vi "choose_crystals.vi"(5 "ROI Size":T2, 7 "Parameters":T3, 8 "Error In":errorcluster, 9 "Xi":T4, 10 "Sample":string, 11 "File Path":path) -> (0 "Error Out":errorcluster, 3 "ROIs Out":T1(array[cluster]))   [LabVIEW 2019]
uses:
  xi_angles_enum_typedef.ctl
  parameters_cluster_typedef.ctl
  sections_roi_size_enum_typedef.ctl
  choose_crystals_states_enum_typedef.ctl
  <vilib>/vision/NI_Vision_Development_Module.lvlib
panel:
  in  "Done":bool
  in  "Frame":i32(slide) scale=0.0..3.0
  in  "X Value":sgl format="%.2f"
  in  "Operator":T5(ring)
  out "Image":T6(plugin-control)
  # "Choose Crystals"
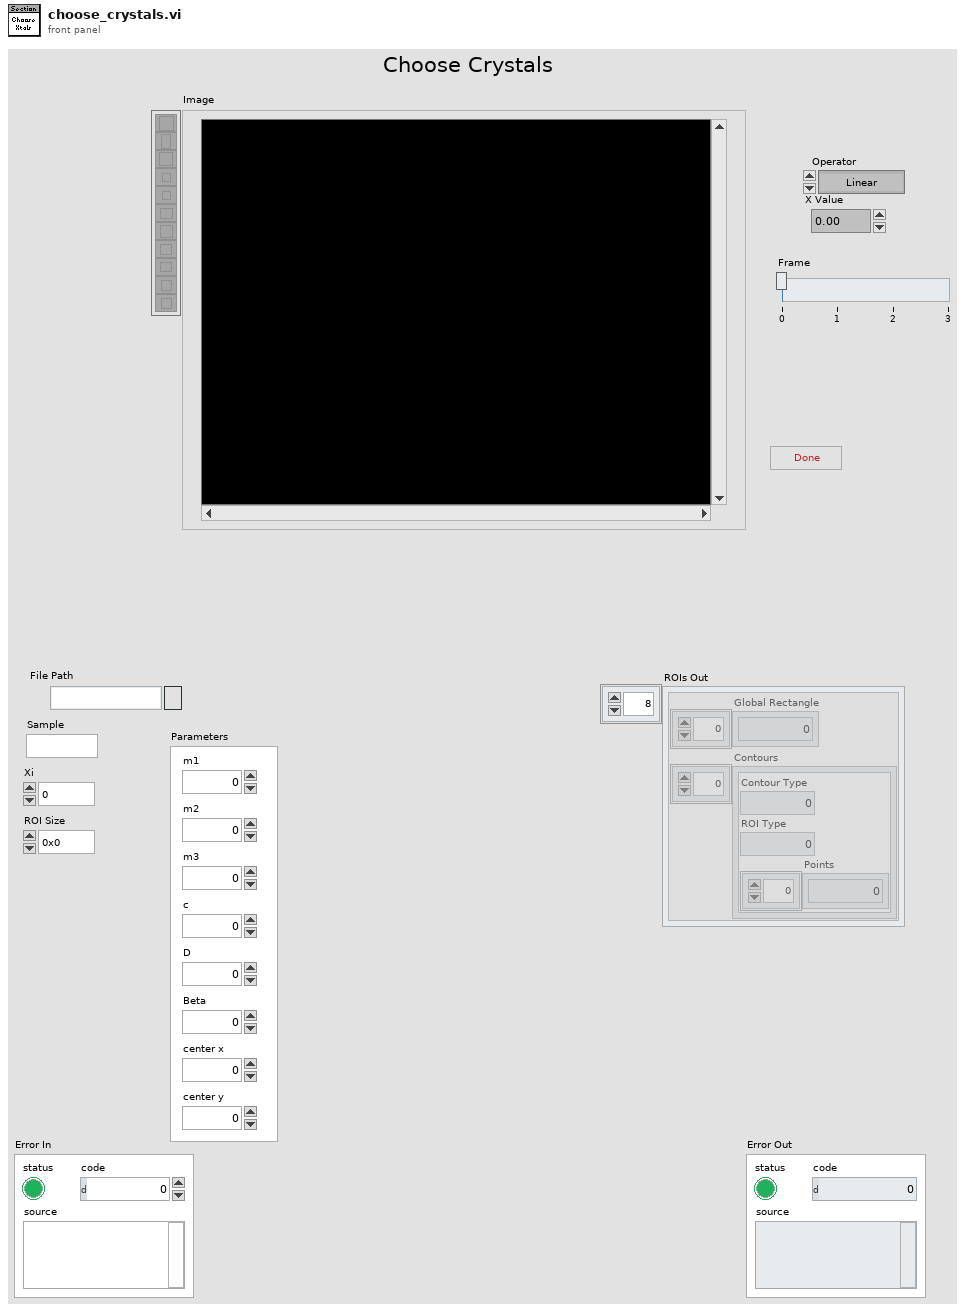
[diagram p1: front panel]
types:
  T1 = cluster{"Global Rectangle":i32[], "Contours":cluster{"Contour Type":u32, "ROI Type":u32, "Points":i32[]}[]}[]
  T2 = typedef "sections_roi_size_enum_typedef.ctl" = enum16{"0x0", "1x1", "2x2", "3x3", "4x4", "5x5", "6x6"}
  T3 = typedef "parameters_cluster_typedef.ctl" = cluster{"m1":dbl, "m2":dbl, "m3":dbl, "c":dbl, "D":dbl, "Beta":dbl, "center x":dbl, "center y":dbl}
  T4 = typedef "xi_angles_enum_typedef.ctl" = enum16{"0", "45"}
  T5 = enum32{"Linear", "Log", "Exp", "Square", "Square root", "Power X", "Power 1/X"}
  T6 = typedef "IMAQ Image.ctl" = refnum<image>
  T7 = typedef "choose_crystals_states_enum_typedef.ctl" = enum16{"Initialize", "Wait", "Shutdown", "Plot Image", "Process"}
  T8 = cluster{"Global Rectangle":i32[], "Contours":cluster{"Contour Type":u32, "ROI Type":u32, "Points":i32[]}[]}
  T9 = typedef "ROI Descriptor" = cluster{"Global Rectangle":i32[], "Contours":cluster{"ID":enum32{"External", "Internal"}, "Type":u32, "Coordinates":i32[]}[]}
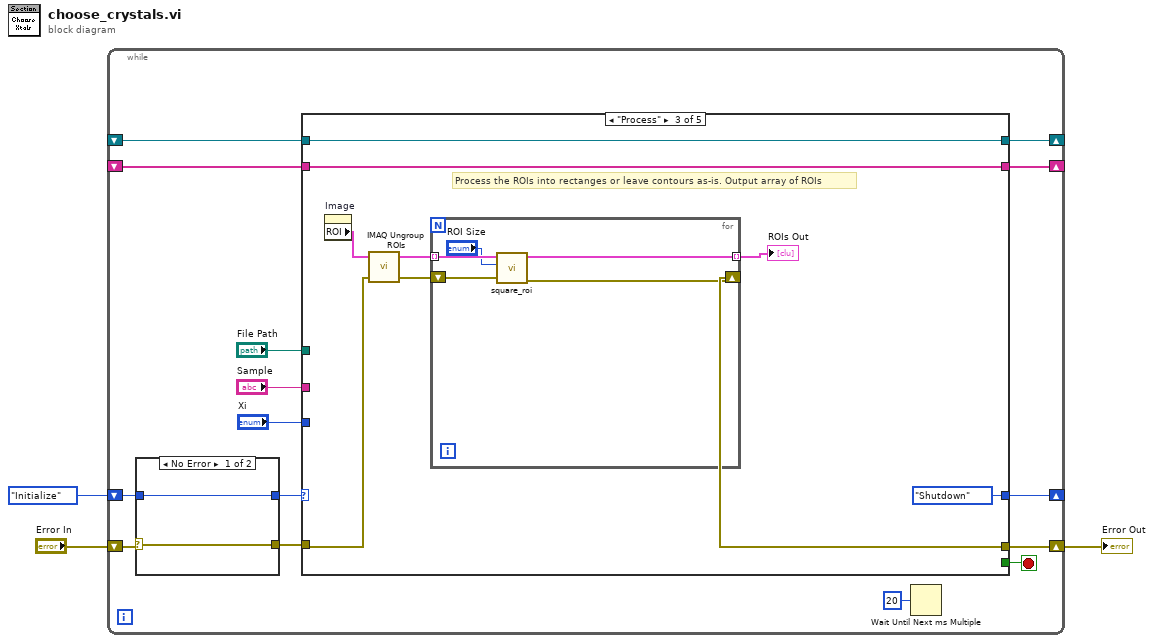
[diagram p0: block diagram]
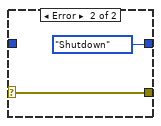
[diagram p2: hidden frame]
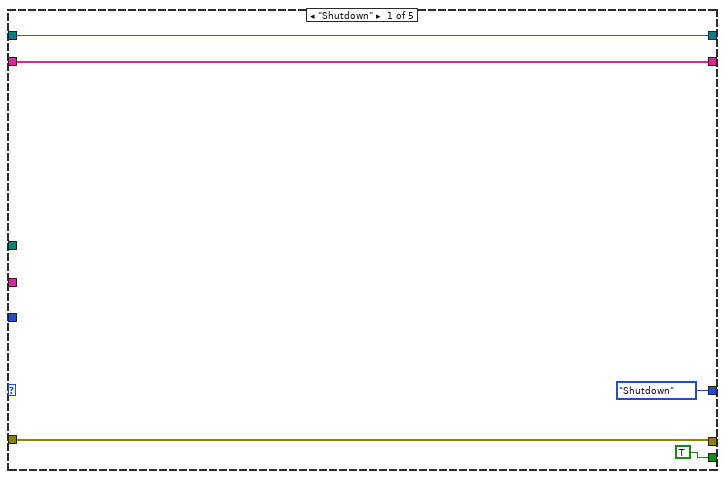
[diagram p3: hidden frame]
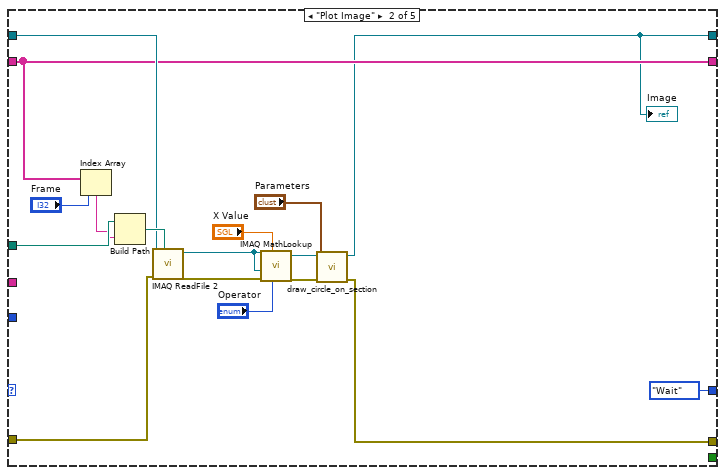
[diagram p4: hidden frame]
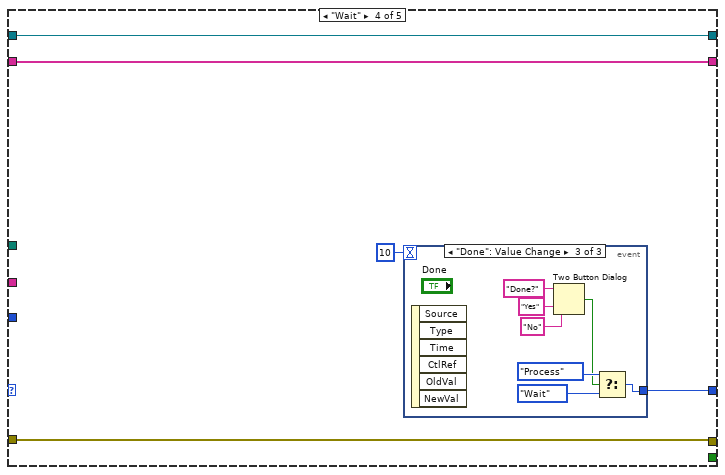
[diagram p5: hidden frame]
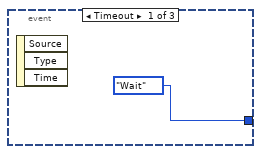
[diagram p6: hidden frame]
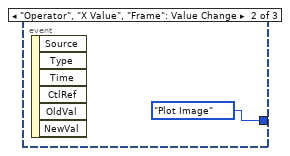
[diagram p7: hidden frame]
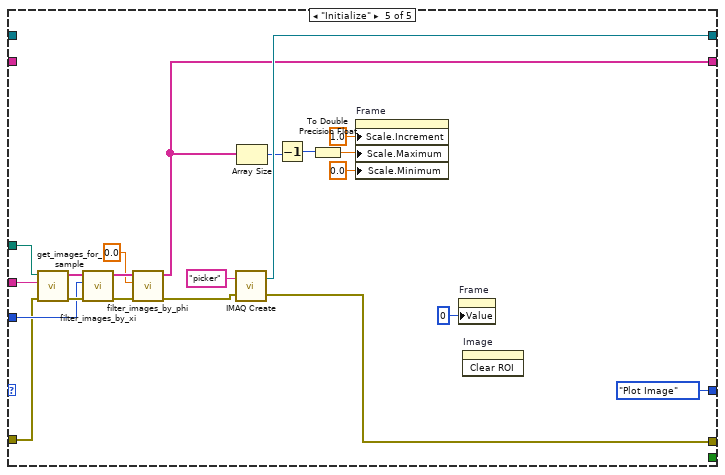
[diagram p8: hidden frame]
diagram:
  n1 = while {
    shift-right: [w14] -> _
    shift-left: choose_crystals_states_enum_typedef."Initialize" -> [w17]
    shift-right: [w13] -> w1
    shift-left: "Error In" -> [w16]
    shift-right: [w7] -> _
    shift-left: _ -> [w6]
    shift-right: [w5] -> _
    shift-left: _ -> [w4]
    stop <- w11 stop-if-true
    n2 = case shown="No Error" w16 {
      selector: w16 -> [w19 w22]
      tunnel: [w20 choose_crystals_states_enum_typedef."Shutdown"] -> w18
      tunnel: w17 -> [w20 _]
      tunnel: [w19 w22] -> w15
      frame No Error {
      }
      frame Error {
      }
    }
    n3 = case shown="\"Process\"" w18 {
      tunnel: w15 -> [w26 w37 w49 w61 w84]
      tunnel: [choose_crystals_states_enum_typedef."Shutdown" choose_crystals_states_enum_typedef."Wait" choose_crystals_states_enum_typedef."Shutdown" w62 choose_crystals_states_enum_typedef."Plot Image"] -> w14
      tunnel: [w26 w29 w45 w61 w83] -> w13
      tunnel: [TRUE _ _ _ _] -> w11
      tunnel: "File Path" -> [_ w40 _ _ w92]
      tunnel: "Sample" -> [_ _ _ _ w91]
      tunnel: "Xi" -> [_ _ _ _ w86]
      tunnel: [w23 w35 w51 w59 w74] -> w7
      tunnel: w6 -> [w23 w35 w51 w59 _]
      tunnel: [w24 w28 w52 w60 w80] -> w5
      tunnel: w4 -> [w24 w36 w52 w60 _]
      frame "Shutdown" {
      }
      frame "Plot Image" {
        n4 = Index Array(array=w35, index="Frame") -> (element=w39:string)
        n5 = Build Path(base path=w40, name or relative path=w39) -> (appended path=w38:path)
        n6 = call "IMAQ ReadFile 2"("File Path"=w38, "error in (no error)"=w37, "Image"=w36) -> ("error out"=w33:errorcluster, "Image Out"=w34:T6)  [unwired: 4 in, 3 out]
        n7 = call "IMAQ MathLookup"("Operator"="Operator", "X Value"="X Value", "error in (no error)"=w33, "Image Dst"=w34, "Image Src"=w34) -> ("error out"=w30:errorcluster, "Image Dst Out"=w32:T6)  [unwired: 5 in]
        n8 = call "draw_circle_on_section.vi"("Error In"=w30, "Parameters"="Parameters", "Image Src"=w32) -> ("Error Out"=w29:errorcluster, "Image Dst Out"=w28:T6)  [unwired: 7 in]
        "Image" <- w28
      }
      frame "Process" {
        # "Process the ROIs into rectanges or leave contours as-is. Output array of ROIs"
        n9 = property on="Image" class="ImageControl"() -> ("ROI"=w50:T8)  [unwired: 2 in, 2 out]
        n10 = call "IMAQ Ungroup ROIs"("error in (no error)"=w49, "ROI Descriptor"=w50) -> ("error out"=w47:errorcluster, "ROI Descriptors out"=w48:T9[])  [unwired: 2 in]
        n11 = for {
          tunnel: w48 -> [w58] mode=indexing
          shift-right: [w55] -> w45
          shift-left: w47 -> [w57]
          tunnel: [w54] -> w46 mode=indexing
          n12 = call "square_roi.vi"("Error In"=w57, "ROI Size"="ROI Size", "ROI In"=w58) -> ("Error Out"=w55:errorcluster, "ROI Out"=w54:T8)  [unwired: 7 in]
        }
        "ROIs Out" <- w46
      }
      frame "Wait" {
        n13 = event shown="[2] \"Done\": Value Change" {
          selector: _ -> [_ _ _]
          dyn-events: _ -> [_ _ _]
          timeout: 10 -> [_ _ _]
          tunnel: [choose_crystals_states_enum_typedef."Wait" choose_crystals_states_enum_typedef."Plot Image" w70] -> w62
          event Timeout {
            n14 = event-data() -> ()  [unwired: 1 in, 3 out]
          }
          event "Operator", "X Value", "Frame": Value Change {
            n15 = event-data() -> ()  [unwired: 1 in, 6 out]
          }
          event "Done": Value Change {
            n16 = event-data() -> ()  [unwired: 1 in, 6 out]
            n17 = Two Button Dialog(message="Done?", 1:"No" ("F button name (\"Cancel\")"), 2:"Yes" ("T button name (\"OK\")")) -> (T button?=w69:bool)
            n18 = Select(t=choose_crystals_states_enum_typedef."Process", s=w69, f=choose_crystals_states_enum_typedef."Wait") -> (s? t:f=w70:T7)
          }
        }
      }
      frame "Initialize" {
        n19 = call "get_images_for_sample.vi"("Error In"=w84, "Sample"=w91, "File Path"=w92) -> ("Error Out"=w90:errorcluster, "Image Names"=w87:string[])  [unwired: 7 in]
        n20 = call "filter_images_by_xi.vi"("Error In"=w90, "Xi"=w86, "Image Names"=w87) -> ("Error Out"=w89:errorcluster, "Filtered Image Names"=w88:string[])  [unwired: 7 in]
        n21 = call "filter_images_by_phi.vi"("Error In"=w89, "Phi"=0.0, "Image Names"=w88) -> ("Error Out"=w82:errorcluster, "Filtered Image Names"=w74:string[])  [unwired: 7 in]
        n22 = call "IMAQ Create"("Image Name"="picker", "error in (no error)"=w82) -> ("New Image"=w80:T6, "error out"=w83:errorcluster)  [unwired: 3 in]
        n23 = Array Size(array=w74) -> (size(s)=w75:i32)
        n24 = Decrement(x=w75) -> (x-1=w76:i32)
        n25 = To Double Precision Float(number=w76) -> (double precision float=w77:dbl)
        n26 = property on="Frame" class="Slide (strict)"("Scale.Increment"=1.0 ("Scale.Range:Increment"), "Scale.Maximum"=w77, "Scale.Minimum"=0.0 ("Scale.Range:Minimum")) -> ()  [unwired: 2 in, 2 out]
        n27 = property on="Frame" class="Slide (strict)"("Value"=0 ("Frame")) -> ()  [unwired: 2 in, 2 out]
        n28 = invoke on="Image" class="ImageControl" method="Clear ROI"() -> ()  [unwired: 3 in, 3 out]
      }
    }
    n29 = Wait Until Next ms Multiple(millisecond multiple=u32 20) -> ()  [unwired: 1 out]
  }
  "Error Out" <- w1
